vi "Shift.vi"(10 "Confirmação":bool, 11 "DataIn":T1={"Quem Joga"="", "Tabuleiro"={"(0,0)"="", "(1,0)"="", "(0,1)"="", "(1,1)"="", "(2,0)"="", "(1,2)"="", "(2,2)"="", "(0,2)"="", "(2,1) "=""}, "GameOption"=enum."Multiplayer local", "Turno"=FALSE, "Player"="", "Player 1"="", "Player 2"="", "Dificuldade"=enum."Easy", "Table"=[], "Row"=0, "Aceitar Convite"=FALSE, "Inviter line"=0, "diretório"=path "", "Logout - panel close"=FALSE, "StartGame"=FALSE, "MatchData.lvclass"=refnum, "GameMode"=enum."Single Easy"}) -> (0 "Turno":string, 1 "Tabuleiro":T2, 3 "DataOut":T1={"Quem Joga"="", "Tabuleiro"={"(0,0)"="", "(1,0)"="", "(0,1)"="", "(1,1)"="", "(2,0)"="", "(1,2)"="", "(2,2)"="", "(0,2)"="", "(2,1) "=""}, "GameOption"=enum."Multiplayer local", "Turno"=FALSE, "Player"="", "Player 1"="", "Player 2"="", "Dificuldade"=enum."Easy", "Table"=[], "Row"=0, "Aceitar Convite"=FALSE, "Inviter line"=0, "diretório"=path "", "Logout - panel close"=FALSE, "StartGame"=FALSE, "MatchData.lvclass"=refnum, "GameMode"=enum."Single Easy"})   [LabVIEW 2018]
doc: "SubVi criada para controlar a troca de turnos entre jogadores durante uma partida."
uses:
  controls/DataIn.ctl
  MatchDataClasses/MatchData/MatchData.lvclass
  controls/Tabuleiro.ctl
  controls/GameOption.ctl
  controls/Table.ctl
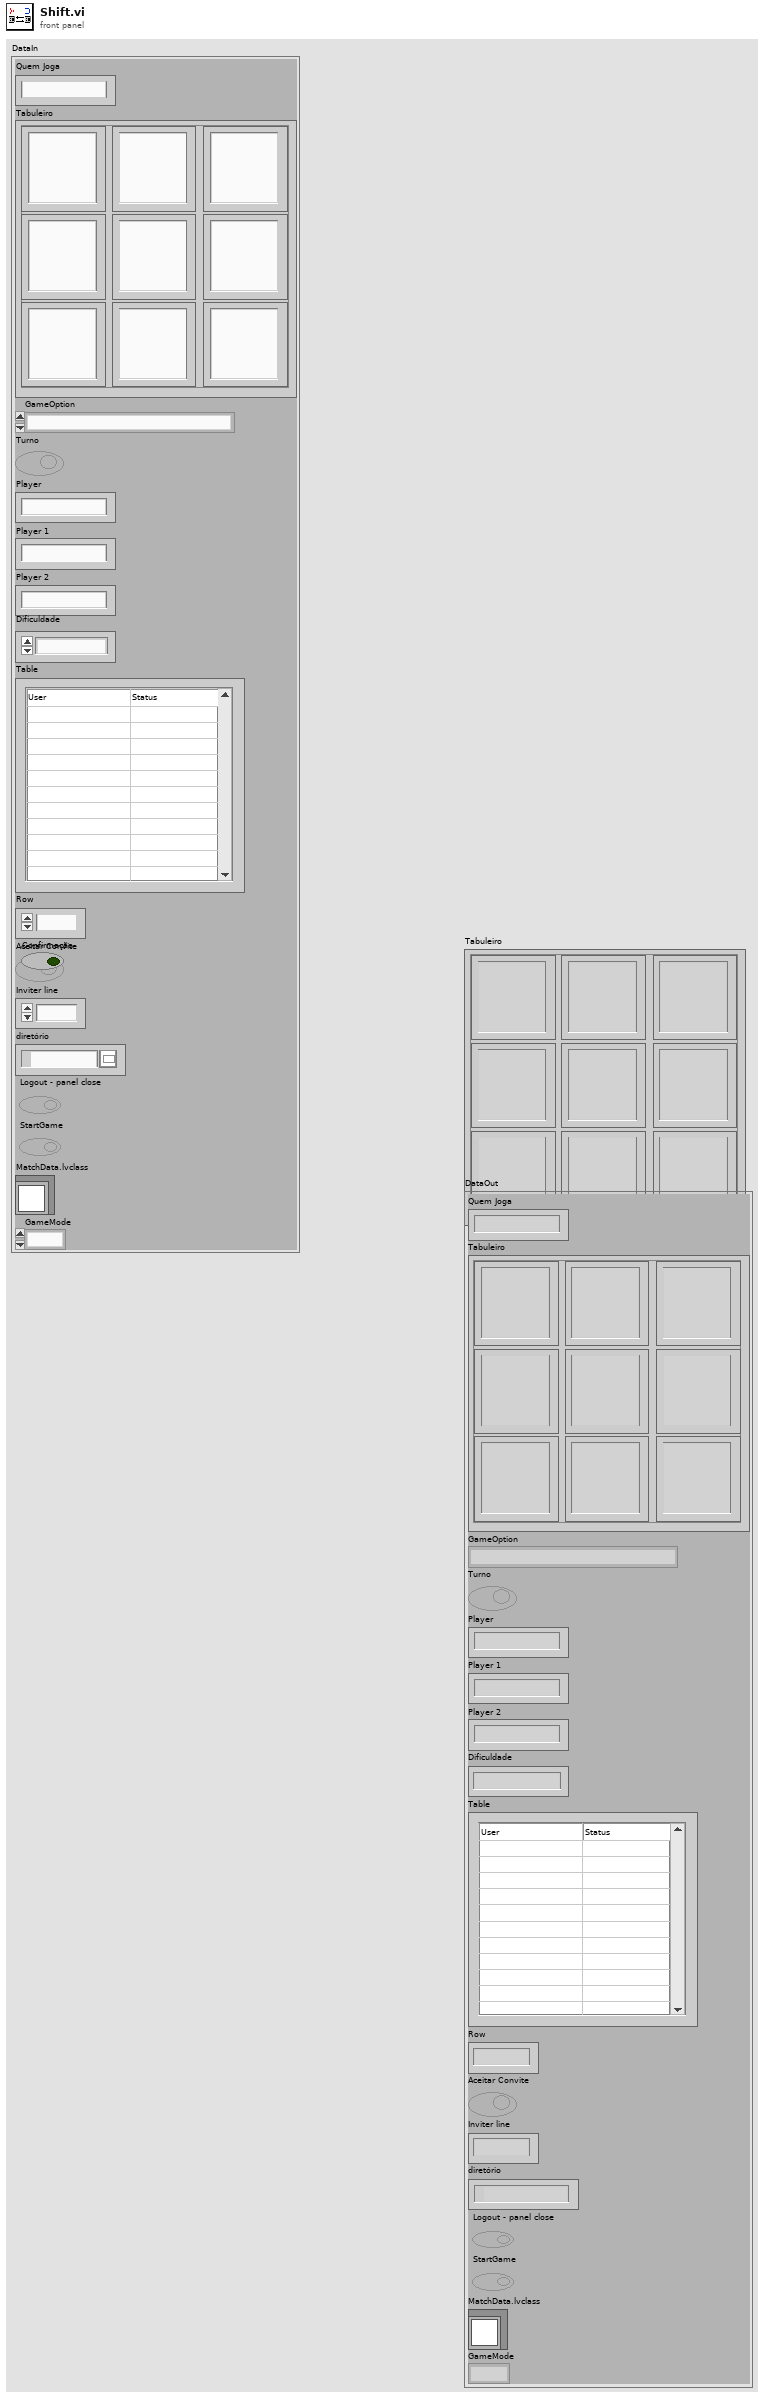
[diagram p1: front panel]
types:
  T1 = typedef "DataIn.ctl" = cluster{"Quem Joga":string, "Tabuleiro":T2, "GameOption":T3, "Turno":bool, "Player":string, "Player 1":string, "Player 2":string, "Dificuldade":enum16{"Easy", "Medium", "Hard"}, "Table":T4, "Row":u32, "Aceitar Convite":bool, "Inviter line":u32, "diretório":path, "Logout - panel close":bool, "StartGame":bool, "MatchData.lvclass":refnum<class "MatchData.lvclass">, "GameMode":enum16{"Single Easy", "Single Medium", "Single Hard", "Local", "Remote"}}
  T2 = typedef "Tabuleiro.ctl" = cluster{"(0,0)":string, "(1,0)":string, "(0,1)":string, "(1,1)":string, "(2,0)":string, "(1,2)":string, "(2,2)":string, "(0,2)":string, "(2,1) ":string}
  T3 = typedef "GameOption.ctl" = enum16{"Single Player", "Multiplayer local", "Multiplayer remoto", "Wait for Event", "Initialize", "Stop"}
  T4 = typedef "Table.ctl" = string[][]
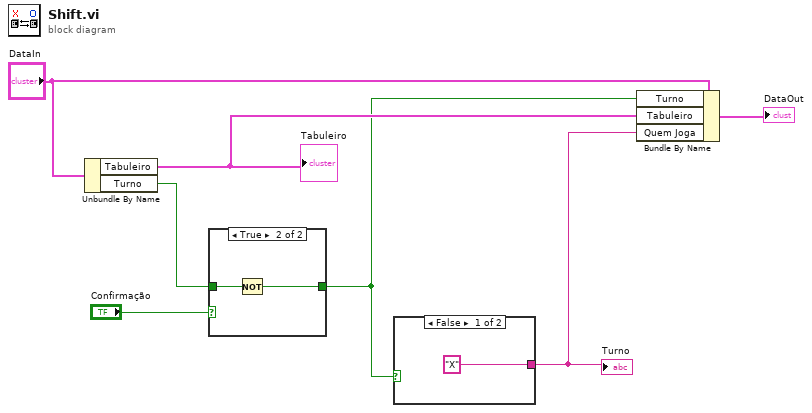
[diagram p0: block diagram]
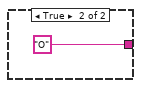
[diagram p2: hidden frame]
diagram:
  n1 = Unbundle By Name("DataIn") -> ("Tabuleiro"=w6:T2, "Turno"=w5:bool)
  "Tabuleiro" <- w6
  n2 = case shown="True" "Confirmação" {
    selector: "Confirmação" -> [w8 _]
    tunnel: [w8 w10] -> w3
    tunnel: w5 -> [_ w9]
    frame False {
    }
    frame True {
      n3 = Not(x=w9) -> (.not. x?=w10:bool)
    }
  }
  n4 = case shown="False" w3 {
    tunnel: ["X" "O"] -> w2
    frame False {
    }
    frame True {
    }
  }
  "Turno" <- w2
  n5 = Bundle By Name(cluster="DataIn", "Turno"=w3, "Tabuleiro"=w6, "Quem Joga"=w2) -> (→"DataOut":T1)
